vi "Downshift MLE Baseline.vi"(0 "Fit Control Data in":T8, 1 "NL Fit Method":T2, 3 "IRF":T1, 5 "rescaled, w sigma":T3={"best nonlinear fit"=[], "best fit parameters"=[], "R^2"=0.0, "RMSE"=0.0, "error out"={"status"=FALSE, "code"=0, "source"=""}, "Fitting Method"=enum."Least Square", "number of function calls"=0, "number of iterations"=0, "covariance"=[], "Chi 2"=0.0, "DOF"=0, "Fit Convergence Criterion"=enum."Continue", "Fitting Algorithm"=enum."Levenberg-Marquardt", "Weighted Fit"=enum."Unweighted", "Gradient"=0.0, "|Delta Chi 2|"=0.0, "|Delta Chi 2|/Chi 2"=0.0, "Max |Delta a| /|a|"=0.0, "Lambda"=-1.0, "RSS"=0.0, "AIC"=0.0, "BIC"=0.0, "Max number of function calls"=0, "Max number of iterations"=0, "IRF"={"X Array"=[], "Y Array"=[]}, "IRF Normalization Factor"=0.0, "Decay Normalization Factor"=0.0, "Number of offset fits"=0, "Weighted Chi2"=-1.0, "Unweighted Chi2"=-1.0}, 7 "Fitted unscaled parameters (w tau)":dbl[](array[numeric]), 9 "All unscaled parameters (w tau)":dbl[](array[numeric]), 11 "All Guess Parameters (w tau)":dbl[](array[numeric]), 12 "MLE_Baseline_Shift":dbl=1.0 format="%#_13g") -> (4 "Fit Control Data out":T8, 6 "Fit Output":T3={"best nonlinear fit"=[], "best fit parameters"=[], "R^2"=0.0, "RMSE"=0.0, "error out"={"status"=FALSE, "code"=0, "source"=""}, "Fitting Method"=enum."Least Square", "number of function calls"=0, "number of iterations"=0, "covariance"=[], "Chi 2"=0.0, "DOF"=0, "Fit Convergence Criterion"=enum."Continue", "Fitting Algorithm"=enum."Levenberg-Marquardt", "Weighted Fit"=enum."Unweighted", "Gradient"=0.0, "|Delta Chi 2|"=0.0, "|Delta Chi 2|/Chi 2"=0.0, "Max |Delta a| /|a|"=0.0, "Lambda"=0.0, "RSS"=0.0, "AIC"=0.0, "BIC"=0.0, "Max number of function calls"=0, "Max number of iterations"=0, "IRF"={"X Array"=[], "Y Array"=[]}, "IRF Normalization Factor"=0.0, "Decay Normalization Factor"=0.0, "Number of offset fits"=0, "Weighted Chi2"=-1.0, "Unweighted Chi2"=-1.0}, 8 "Fitted unscaled parameters (w tau)":dbl[](array[numeric]), 10 "All unscaled Parameters (w tau)":dbl[](array[numeric]), 15 "All Guess Parameters (w tau)":dbl[](array[numeric]))   [LabVIEW 2021, in "Fits.lvlib"]
uses:
  Fits.lvlib
  Decay Convolution/Fit Control Data v2.ctl
  Graphs/XY Graph/XY Graph Plot Data.ctl
  Decay Fit Parameters In List.ctl
  Decay Convolution/Decay Model.ctl
  Non-linear Fit Output v4.ctl
  Nonlinear Fit Method.ctl
  <vilib>/Analysis/Matrix/Datatypes/RealMatrix.ctl
  Convergence Criteria.ctl
  Non-linear Fitting Algorithm.ctl
  Fit Weights Type v2.ctl
  Graphs/XY Graph/XY Graph Add-Ons.lvlib
  <vilib>/Analysis/Matrix/NI_Matrix.lvlib
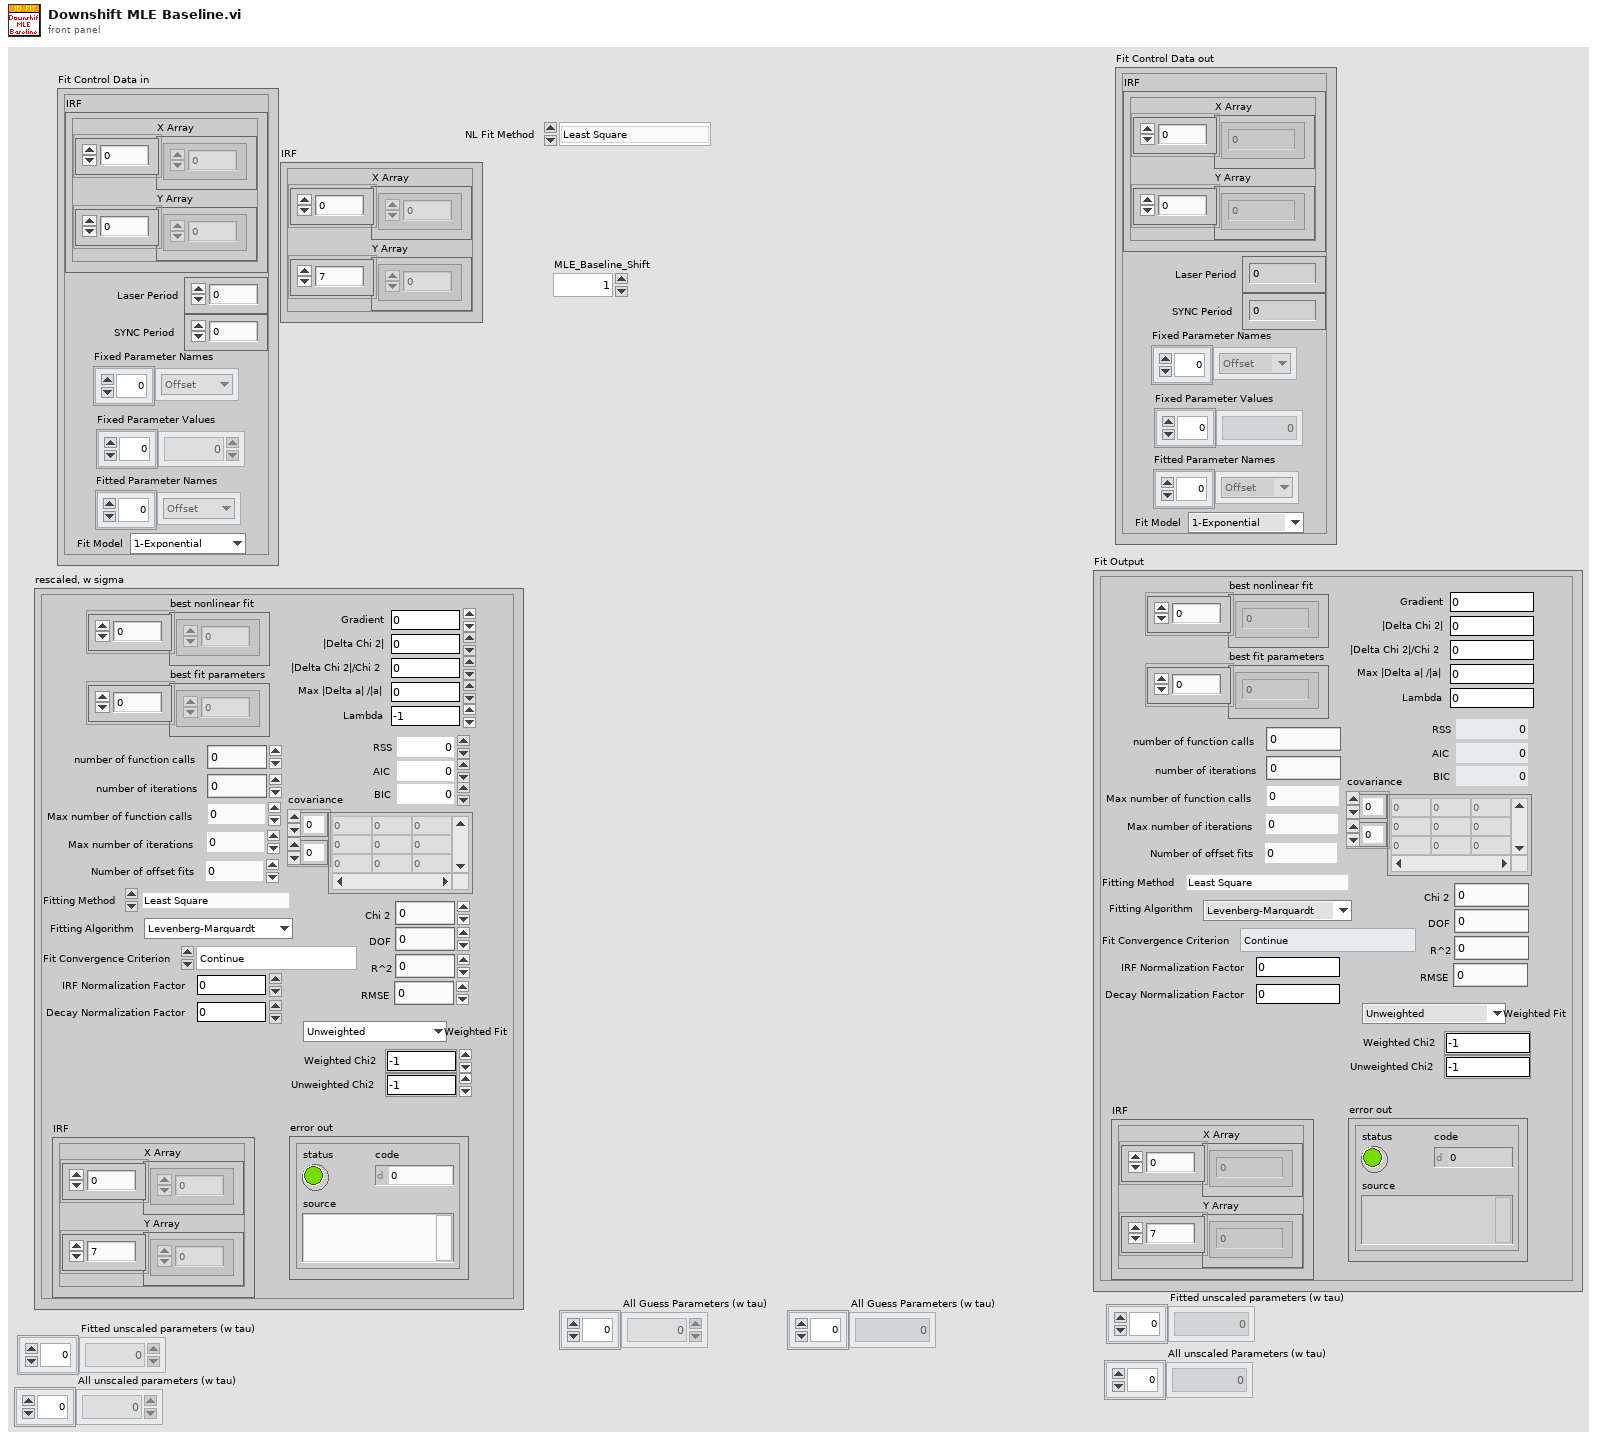
[diagram p1: front panel]
types:
  T1 = typedef "XY Graph Add-Ons.lvlib/XY Graph Plot Data.ctl" = cluster{"X Array":dbl[], "Y Array":dbl[]}
  T2 = typedef "Fits.lvlib/Nonlinear Fit Method.ctl" = enum16{"Least Square", "Least Absolute Residual", "Bisquare", "MLE"}
  T3 = typedef "Fits.lvlib/Non-linear Fit Output v4.ctl" = cluster{"best nonlinear fit":dbl[], "best fit parameters":dbl[], "R^2":dbl, "RMSE":dbl, "error out":errorcluster, "Fitting Method":T2, "number of function calls":i32, "number of iterations":i32, "covariance":T4, "Chi 2":dbl, "DOF":i32, "Fit Convergence Criterion":T5, "Fitting Algorithm":T6, "Weighted Fit":T7, "Gradient":dbl, "|Delta Chi 2|":dbl, "|Delta Chi 2|/Chi 2":dbl, "Max |Delta a| /|a|":dbl, "Lambda":dbl, "RSS":dbl, "AIC":dbl, "BIC":dbl, "Max number of function calls":i32, "Max number of iterations":i32, "IRF":T1, "IRF Normalization Factor":dbl, "Decay Normalization Factor":dbl, "Number of offset fits":i32, "Weighted Chi2":dbl, "Unweighted Chi2":dbl}
  T4 = typedef "NI_Matrix.lvlib/RealMatrix.ctl" = dbl[][]
  T5 = typedef "Fits.lvlib/Convergence Criteria.ctl" = enum16{"Continue", "Tolerances Exceeded", "Max Time Exceeded", "Max Iterations Exceeded", "Max Function Evaluations Exceeded", "Scale Range Exceeded"}
  T6 = typedef "Fits.lvlib/Non-linear Fitting Algorithm.ctl" = enum16{"Levenberg-Marquardt", "Trust-Region Dogleg"}
  T7 = typedef "Fits.lvlib/Fit Weights Type v2.ctl" = enum16{"Unweighted", "1/Variance (Neyman)", "1/Variance (Pearson)", "Best of All"}
  T8 = typedef "Fits.lvlib/Fit Control Data v2.ctl" = cluster{"IRF":T1, "Laser Period":dbl, "SYNC Period":dbl, "Fixed Parameter Names":T9[], "Fixed Parameter Values":dbl[], "Fitted Parameter Names":T9[], "Fit Model":T10}
  T9 = typedef "Fits.lvlib/Decay Fit Parameters In List.ctl" = enum16{"Offset", "Baseline", "A_1", "tau_1", "A_2", "tau_2"}
  T10 = typedef "Fits.lvlib/Decay Model.ctl" = enum16{"1-Exponential", "2-Exponentials"}
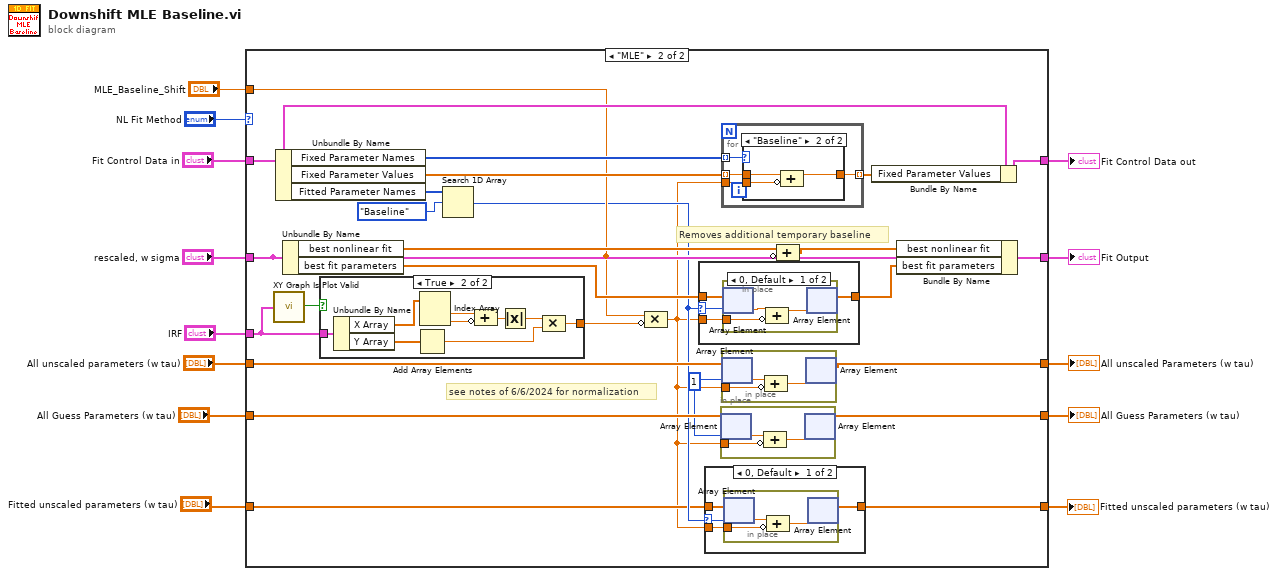
[diagram p0: block diagram]
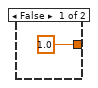
[diagram p4: hidden frame]
diagram:
  n1 = case shown="\"MLE\"" "NL Fit Method" {
    tunnel: "Fit Control Data in" -> [w18 w42]
    tunnel: "rescaled, w sigma" -> [w17 w37]
    tunnel: "All unscaled parameters (w tau)" -> [w16 w33]
    tunnel: "All Guess Parameters (w tau)" -> [w15 w31]
    tunnel: [w18 w40] -> w8
    tunnel: [w17 w34] -> w7
    tunnel: [w16 w32] -> w6
    tunnel: [w15 w29] -> w5
    tunnel: "MLE_Baseline_Shift" -> [_ w25]
    tunnel: "IRF" -> [_ w24]
    tunnel: "Fitted unscaled parameters (w tau)" -> [w14 w21]
    tunnel: [w14 w20] -> w1
    frame "Least Square", Default {
    }
    frame "MLE" {
      w30 = 1
      # "Removes additional temporary baseline"
      # "see notes of 6/6/2024 for normalization"
      n2 = call "XY Graph Is Plot Valid.vi"("Plot"=w24) -> ("Is Valid Plot?"=w23:bool)  [unwired: 8 in]
      n3 = Unbundle By Name(w42) -> ("Fixed Parameter Names"=w44:T9[], "Fixed Parameter Values"=w43:dbl[], "Fitted Parameter Names"=w28:T9[])
      n4 = Unbundle By Name(w37) -> ("best nonlinear fit"=w39:dbl[], "best fit parameters"=w38:dbl[])
      n5 = case shown="True" w23 {
        tunnel: [1.0 w57] -> w26
        tunnel: w24 -> [_ w56]
        frame False {
        }
        frame True {
          n6 = Unbundle By Name(w56) -> ("X Array"=w55:dbl[], "Y Array"=w54:dbl[])
          n7 = Add Array Elements(numeric array=w54) -> (sum=w58:dbl)
          n8 = Index Array(array=w55) -> (element #1=w62:dbl, element #2=w61:dbl)  [unwired: 2 in]
          n9 = Compound Arithmetic op=ADD(w62, invert w61) -> (w60:dbl)
          n10 = Absolute Value(x=w60) -> (abs(x)=w59:dbl)
          n11 = Compound Arithmetic op=MULTIPLY(w59, w58) -> (w57:dbl)
        }
      }
      n12 = Search 1D Array(1D array=w28, element=Decay_Fit_Parameters_In_List."Baseline") -> (index of element=w22:i32)  [unwired: 1 in]
      n13 = Compound Arithmetic op=MULTIPLY(w25, invert w26) -> (w19:dbl)
      n14 = case shown="0, Default" w22 {
        selector: w22 -> [w63 _]
        tunnel: w38 -> [w66 w70]
        tunnel: [w65 w70] -> w35
        tunnel: w19 -> [w64 _]
        frame 0, Default {
          n15 = in-place {
            in-place-border: w64 -> [w67]
            n16 = in-place-array #1(w66, w63) -> (w69:dbl)
            n17 = Compound Arithmetic op=ADD(w69, invert w67) -> (w68:dbl)
            n18 = in-place-array #1(w68) -> (w65:dbl[])  [unwired: 1 out]
          }
        }
        frame -1 {
        }
      }
      n19 = case shown="0, Default" w22 {
        selector: w22 -> [w48 _]
        tunnel: w21 -> [w47 w52]
        tunnel: [w46 w52] -> w20
        tunnel: w19 -> [w45 _]
        frame 0, Default {
          n20 = in-place {
            in-place-border: w45 -> [w49]
            n21 = in-place-array #2(w47, w48) -> (w51:dbl)
            n22 = Compound Arithmetic op=ADD(w51, invert w49) -> (w50:dbl)
            n23 = in-place-array #2(w50) -> (w46:dbl[])  [unwired: 1 out]
          }
        }
        frame -1 {
        }
      }
      n24 = in-place {
        in-place-border: w19 -> [w71]
        n25 = in-place-array #3(w31, w30) -> (w73:dbl)
        n26 = Compound Arithmetic op=ADD(w73, invert w71) -> (w72:dbl)
        n27 = in-place-array #3(w72) -> (w29:dbl[])  [unwired: 1 out]
      }
      n28 = for {
        tunnel: w44 -> [w80] mode=indexing
        tunnel: w43 -> [w79] mode=indexing
        tunnel: [w78] -> w41 mode=indexing
        tunnel: w19 -> [w77]
        n29 = case shown="\"Baseline\"" w80 {
          tunnel: w79 -> [w81 w84]
          tunnel: [w81 w83] -> w78
          tunnel: w77 -> [_ w82]
          frame "Offset", Default {
          }
          frame "Baseline" {
            n30 = Compound Arithmetic op=ADD(w84, invert w82) -> (w83:dbl)
          }
        }
      }
      n31 = in-place {
        in-place-border: w19 -> [w74]
        n32 = in-place-array #4(w33, w30) -> (w76:dbl)
        n33 = Compound Arithmetic op=ADD(w76, invert w74) -> (w75:dbl)
        n34 = in-place-array #4(w75) -> (w32:dbl[])  [unwired: 1 out]
      }
      n35 = Compound Arithmetic op=ADD(w39, invert w25) -> (w36:dbl[])
      n36 = Bundle By Name(cluster=w42, "Fixed Parameter Values"=w41) -> (w40:T8)
      n37 = Bundle By Name(cluster=w37, "best nonlinear fit"=w36, "best fit parameters"=w35) -> (w34:T3)
    }
  }
  "Fit Control Data out" <- w8
  "All Guess Parameters (w tau)" <- w5
  "All unscaled Parameters (w tau)" <- w6
  "Fit Output" <- w7
  "Fitted unscaled parameters (w tau)" <- w1
